vi "LIMELIGHT SET.vi"(0 "ledMode":T3 items=["default to current pipeline", "force off", "force blink", "force on"], 1 "camMode":T2 items=["Vision processor", "Driver Camera"], 2 "pipeline":u16(ring) items=["0", "1", "2", "3", "4", "5", "6", "7", "8", "9"], 3 "stream":T1 items=["standard side-by-side", "PiP Main", "PiP Secondary"], 5 "error in (no error)":errorcluster) -> (19 "error out":errorcluster)   [LabVIEW 2023]
uses:
  ctrl defs/ctrl LIMELIGHT LEDMODE selector.ctl
  ctrl defs/ctrl LIMELIGHT CAMMODE selector.ctl
  ctrl defs/ctrl LIMELIGHT STREAM selector.ctl
  <vilib>/Rock Robotics/Network Tables/NT Write Integer.vi
panel:
  in  "snapshot":u16(ring) items=["reset snapshot mode", "take one snapshot"]
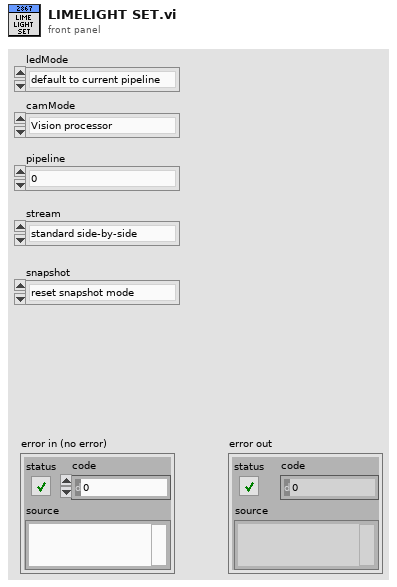
[diagram p1: front panel]
types:
  T1 = typedef "ctrl LIMELIGHT STREAM selector.ctl" = u16
  T2 = typedef "ctrl LIMELIGHT CAMMODE selector.ctl" = u16
  T3 = typedef "ctrl LIMELIGHT LEDMODE selector.ctl" = u16
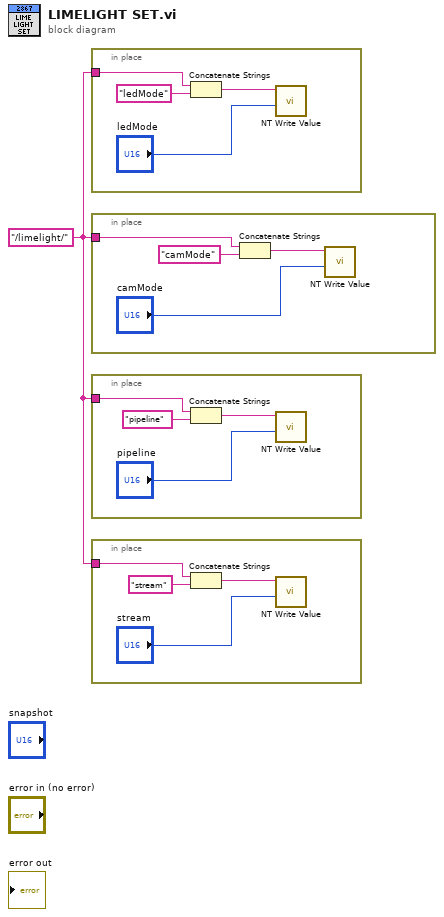
[diagram p0: block diagram]
diagram:
  w1 = "/limelight/"
  n1 = in-place {
    in-place-border: w1 -> [w2]
    n2 = Concatenate Strings(w2, "ledMode") -> (w4:string)
    n3 = call-poly <vilib>:"NT Write Value.vi"("value"="ledMode", "name"=w4) -> ()  [unwired: 9 in, 1 out]
  }
  n4 = in-place {
    in-place-border: w1 -> [w6]
    n5 = Concatenate Strings(w6, "camMode") -> (w8:string)
    n6 = call-poly <vilib>:"NT Write Value.vi"("value"="camMode", "name"=w8) -> ()  [unwired: 9 in, 1 out]
  }
  n7 = in-place {
    in-place-border: w1 -> [w10]
    n8 = Concatenate Strings(w10, "pipeline") -> (w12:string)
    n9 = call-poly <vilib>:"NT Write Value.vi"("value"="pipeline", "name"=w12) -> ()  [unwired: 9 in, 1 out]
  }
  n10 = in-place {
    in-place-border: w1 -> [w14]
    n11 = Concatenate Strings(w14, "stream") -> (w16:string)
    n12 = call-poly <vilib>:"NT Write Value.vi"("value"="stream", "name"=w16) -> ()  [unwired: 9 in, 1 out]
  }
